vi "OE1201_Configure Input Filter.vi"(7 "OE1201_Configure Input Filter":T1 {"Input Notch Filter" items=["None", "50Hz", "100Hz", "Both"]; "Input Coupling" items=["AC", "DC"]; "Input Shield Grounding" items=["Float", "Ground"]; "Input Source" items=["A", "B", "I-1M", "I-100M"]}, 8 "Error in (no error)":errorcluster caption="error out（no error）", 9 "Remote Mode":u16(ring) items=["USB", "RS232"], 11 "VISA resource name":refnum<visa-resource-name>) -> (0 "Error out":errorcluster caption="error out", 1 "Output String":string, 3 "VISA resource  out":refnum<visa-resource-name>)   [LabVIEW 2011]
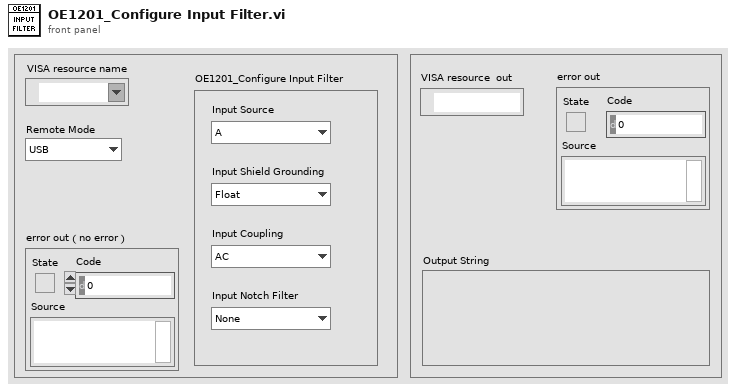
[diagram p1: front panel]
types:
  T1 = cluster{"Input Source":u16, "Input Shield Grounding ":u16, "Input Coupling ":u16, "Input Notch Filter ":u16}
  T2 = enum16{"ISRC", "IGND", "ICPL", "ILIN", "PHAS", "FMOD", "RSLP", "FREQ", "SWPT", "SLLM", "SULM", "SSLL", "SSLG", "STLM", "SWRM", "IRNG", "SENS", "RMOD", "OFLT", "OFSL", "SYNC", "DMOD", "HARM", "DARB", "SWVT", "SLVL", "SVLL", "SVUL", "SVSL", "SVSG", "SVTM", "SVRM", "RALL", "SNAP", "OUTP", "OAUX", "COUT", "CAUX", "COFP", "CEXP", "FPOP", "OEXP", "*IDN", "*RST", "OVLD", "INOV", "GNOV", "*PLL", "SSET", "RSET", "AGAN", "APHS", "ARSV", "ASCL", "EQCD", "EQCS", "SPED", "SRAT", "SLEN", "SSLE", "STRG", "SPRM", "STRD", "PAUS", "REST", "SPTS", "TRCA", "TEMP", "RSTU", "IHNZ", "DEQU", "SADD", "ARNG", "CSPE", "ISRCD", "IGNDD", "ICPLD", "ILIND", "PHASD", "FMODD", "RSLPD", "FREQD", "SWPTD", "SLLMD", "SULMD", "SSLLD", "SSLGD", "STLMD", "SWRMD", "SENSD", "RMODD", "OFLTD", "OFSLD", "SYNCD", "HARMD", "EQCDD", "EQCSD", "SNAPD", "OUTPD", "SWVTD", "SLVLD", "SVLLD", "SVULD", "SVSLD", "SVSGD", "SVTMD", "SVRMD", "SVDCD", "ARSVD", "AGAND", "APHSD", "ASCLD", "FPOPD", "CAUXD", "OEXPD", "SPEDD", "SRATD", "SLEND", "SSLED", "STRGD", "SPRMD", "STRDD", "PAUSD", "RESTD", "SPTSD", "TRCAD", "*IDND", "*RSTD", "INOVD", "GNOVD", "*PLLD", "SSETD", "RSETD"}
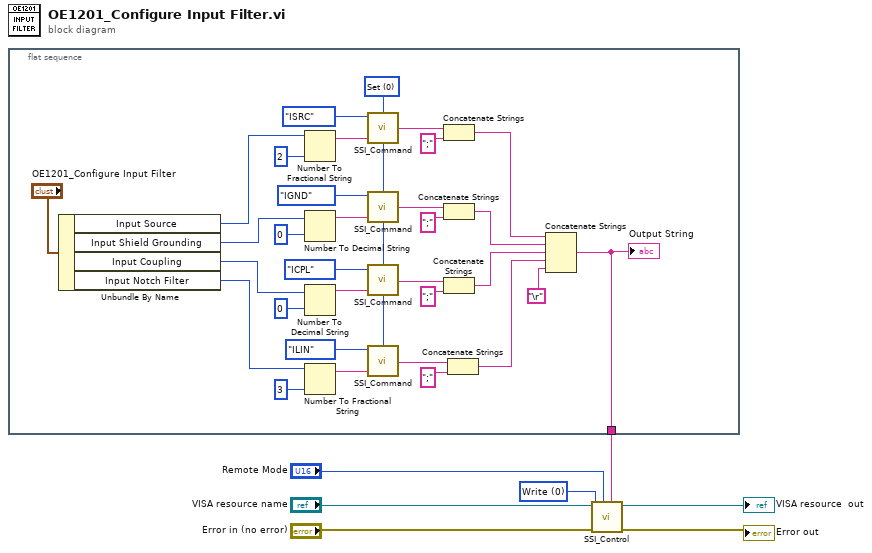
[diagram p0: block diagram]
diagram:
  w6 = u16 0 items=["Write", "Read"] ("Control")
  n1 = flat-sequence {
    tunnel: [w16] -> w1
    frame #0 {
      w17 = u16 0 items=["Set", "Query"] ("Opera")
      n2 = Unbundle By Name("OE1201_Configure Input Filter") -> ("Input Source"=w11:u16, "Input Shield Grounding"=w10:u16, "Input Coupling"=w9:u16, "Input Notch Filter"=w8:u16)
      n3 = Number To Fractional String(number=w11, precision (6)=i16 2 ("精度(6)")) -> (F-format string=w38:string)  [unwired: 2 in]
      n4 = Number To Decimal String(number=w10, width (-)=i16 0 ("精度(6)")) -> (decimal integer string=w35:string)
      n5 = Number To Decimal String(number=w9, width (-)=i16 0 ("精度(6)")) -> (decimal integer string=w32:string)
      n6 = Number To Fractional String(number=w8, precision (6)=i16 3 ("精度(6)")) -> (F-format string=w29:string)  [unwired: 2 in]
      n7 = call "SSI_Command.vi"("Opera"=w17, "Paramter"=w38, "Command Type"=T2."ISRC") -> ("Output string"=w22:string)  [unwired: 1 in]
      n8 = call "SSI_Command.vi"("Opera"=w17, "Paramter"=w35, "Command Type"=T2."IGND") -> ("Output string"=w26:string)  [unwired: 1 in]
      n9 = call "SSI_Command.vi"("Opera"=w17, "Paramter"=w32, "Command Type"=T2."ICPL") -> ("Output string"=w20:string)  [unwired: 1 in]
      n10 = call "SSI_Command.vi"("Opera"=w17, "Paramter"=w29, "Command Type"=T2."ILIN") -> ("Output string"=w24:string)  [unwired: 1 in]
      n11 = Concatenate Strings(w22, ";" ("替换字符串(\"\")")) -> (w19:string)
      n12 = Concatenate Strings(w26, ";" ("替换字符串(\"\")")) -> (w18:string)
      n13 = Concatenate Strings(w20, ";" ("替换字符串(\"\")")) -> (w14:string)
      n14 = Concatenate Strings(w24, ";" ("替换字符串(\"\")")) -> (w13:string)
      n15 = Concatenate Strings(w19, w18, w14, w13, "\r") -> (w16:string)
      "Output String" <- w16
    }
  }
  n16 = call "SSI_Control.vi"("Write Buffer"=w1, "Remote Mode"="Remote Mode", "Error in (no error)"="Error in (no error)", "Control"=w6, "VISA resource name"="VISA resource name") -> ("Error out"=→"Error out":errorcluster, "VISA resource  out"=→"VISA resource  out":refnum<visa-resource-name>)  [unwired: 3 in, 2 out]
